vi "Unix To LV Timestamp.vi"(8 "error in (no error)":errorcluster, 11 "UTC Unix Offset":u64) -> (0 "error out":errorcluster, 3 "TimeStamp":timestamp)   [LabVIEW 2017]
doc: "Converts a unix timestamp (e.g 1000 or 1657389311770) to a labview timestamp (e.g. 01-Jan-1970 02:00:01+02 or 09-July-2022 19:55:11+02)"
panel:
  out "Offset Between Epochs":u64
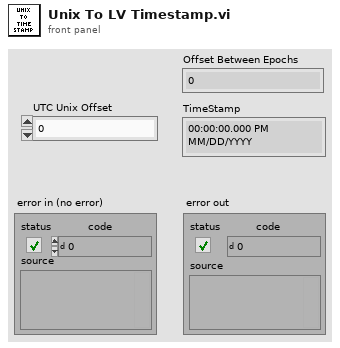
[diagram p1: front panel]
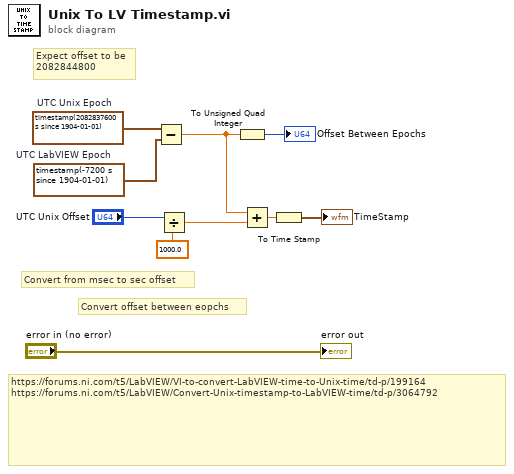
[diagram p0: block diagram]
diagram:
  w8 = timestamp(-7200 s since 1904-01-01)  # UTC LabVIEW Epoch
  w9 = timestamp(2082837600 s since 1904-01-01)  # UTC Unix Epoch
  # "https://forums.ni.com/t5/LabVIEW/VI-to-convert-LabVIEW-time-to-Unix-time/td-p/199164\nhttps://forums.ni.com/t5/LabVIEW/Convert-Unix-timestamp-to-LabVIEW-time/td-p/3064792"
  # "Convert offset between eopchs"
  # "Convert from msec to sec offset"
  # "Expect offset to be\n2082844800"
  n1 = Subtract(x=w9, y=w8) -> (x-y=w4:dbl)
  n2 = Divide(x="UTC Unix Offset", y=1000.0) -> (x/y=w2:dbl)
  n3 = To Unsigned Quad Integer(1:w4) -> (0:→"Offset Between Epochs":u64)
  n4 = Add(x=w4, y=w2) -> (x+y=w6:dbl)
  n5 = To Time Stamp(1:w6) -> (0:→"TimeStamp":timestamp)
  "error out" <- "error in (no error)"
